vi "Generate Content-Type.vi"(11 "Filename":string) -> (3 "Content-Type":string)   [LabVIEW 2019, in "HTTP Server.lvlib"]
uses:
  HTTP Server.lvlib
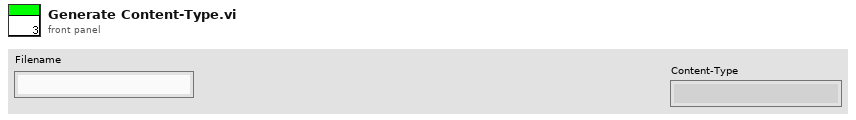
[diagram p1: front panel]
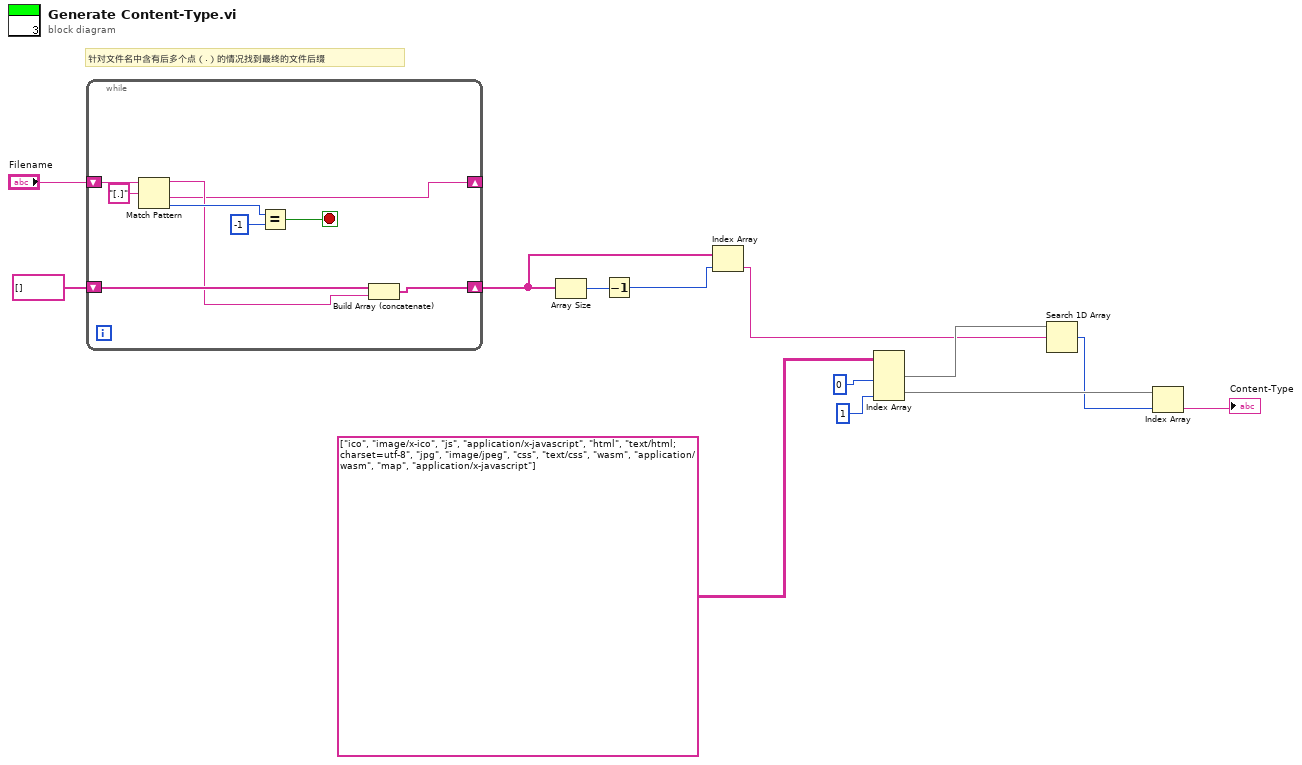
[diagram p0: block diagram]
diagram:
  # "针对文件名中含有后多个点（.）的情况找到最终的文件后缀"
  n1 = while {
    shift-right: [w14] -> _
    shift-left: "Filename" -> [w21]
    shift-right: [w15] -> w4
    shift-left: string[] [] -> [w17]
    stop <- w18 stop-if-true
    n2 = Match Pattern(string=w21, regular expression="[.]" ("正则表达式")) -> (before substring=w16:string, after substring=w14:string, offset past match=w20:i32)  [unwired: 1 in, 1 out]
    n3 = Equal?(x=w20, y=-1) -> (x = y?=w18:bool)
    n4 = Build Array (concatenate)(w17, w16) -> (w15:string[])
  }
  n5 = Array Size(array=w4) -> (size(s)=w3:i32)
  n6 = Decrement(x=w3) -> (x-1=w2:i32)
  n7 = Index Array(array=w4, index=w2) -> (element=w1:string)
  n8 = Index Array(array=string[][] [["ico", "image/x-ico"], ["js", "application/x-javascript"], ["html", "text/html; charset=utf-8"], ["jpg", "image/jpeg"], ["css", "text/css"], ["wasm", "application/wasm"], ["map", "application/x-javascript"]], index (col) #1=0 ("索引 (行)"), index (col) #2=1 ("索引 (列)")) -> (element #1=w10:string[], element #2=w9:string[])  [unwired: 2 in]
  n9 = Search 1D Array(1D array=w10, element=w1) -> (index of element=w8:i32)  [unwired: 1 in]
  n10 = Index Array(array=w9, index=w8) -> (element=→"Content-Type":string)
